vi "SBA-5_initialize.vi"(8 "error in (no error)":errorcluster, 9 "Valve control":bool=TRUE, 11 "VISA resource name":refnum<visa-resource-name>) -> (0 "error out":errorcluster, 3 "VISA resource name out":refnum<visa-resource-name>)   [LabVIEW 2016]
uses:
  <vilib>/Instr/_visa.llb/VISA Flush IO Buffer Mask.ctl
  <vilib>/Instr/_visa.llb/VISA Configure Serial Port (Instr).vi
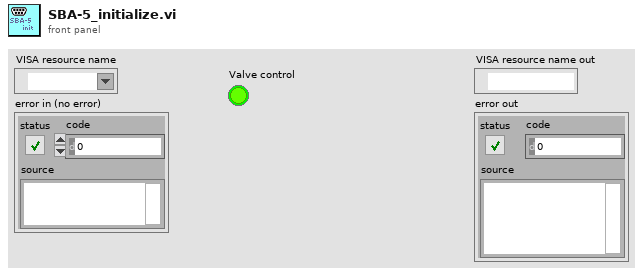
[diagram p1: front panel]
types:
  T1 = typedef "VISA Flush IO Buffer Mask.ctl" = u16
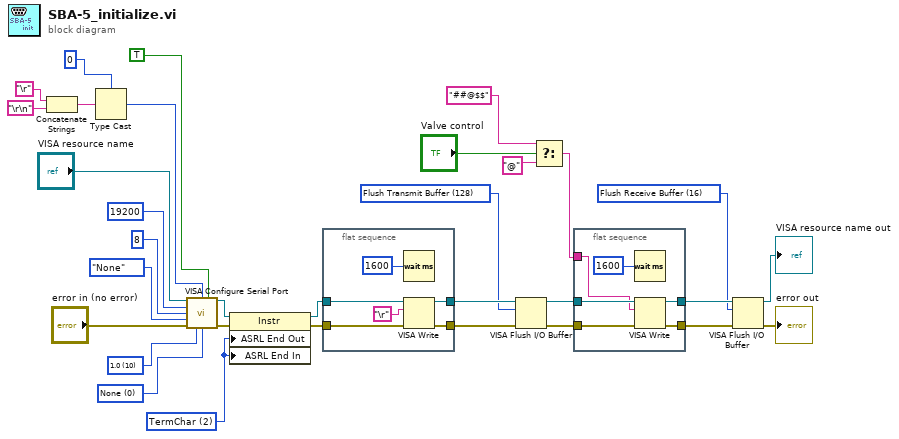
[diagram p0: block diagram]
diagram:
  w5 = T1 16 items=["Flush Receive Buffer"=16, "Write Transmit Buffer to Device"=32, "Flush Receive Buffer (No I/O)"=64, "Flush Transmit Buffer"=128] ("Mask")
  w11 = T1 128 items=["Flush Receive Buffer"=16, "Write Transmit Buffer to Device"=32, "Flush Receive Buffer (No I/O)"=64, "Flush Transmit Buffer"=128] ("Mask")
  w25 = u16 2 items=["None", "Last Bit", "TermChar", "Break"] ("Serial Settings:End Mode for Writes")
  w28 = u16 0 items=["None", "XON/XOFF", "RTS/CTS", "XON/XOFF & RTS/CTS", "DTR/DSR", "XON/XOFF & DTR/DSR"] ("flow control (0:none)")
  w29 = u16 10 items=["1.0"=10, "1.5"=15, "2.0"=20] ("stop bits (10: 1 bit)")
  n1 = Concatenate Strings("\r", "\r\n") -> (w10:string)
  n2 = Type Cast(type=u8 0, x=w10) -> (*(type *) &x=w7:u8)
  n3 = call-poly "VISA Configure Serial Port"("VISA resource name"="VISA resource name", "termination char\n(0xA = '\\n' = LF)"=w7, "Enable Termination\nChar (T)"=TRUE ("Enable Termination\nChar (T)"), "baud rate (9600)"=u32 19200 ("baud rate (19200)"), "data bits (8)"=u16 8, "parity (0:none)"=enum16{"None", "Odd", "Even", "Mark", "Space"}."None", "error in (no error)"="error in (no error)", "stop bits (10: 1 bit)"=w29, "flow control (0:none)"=w28) -> ("VISA resource name out"=w27:refnum<visa-resource-name>, "error out"=w26:errorcluster)  [unwired: 5 in]
  n4 = property class="Instr"(reference=w27, error in=w26, "ASRL End Out"=w25, "ASRL End In"=w25) -> (reference out=w24:refnum<visa-resource-name>, error out=w23:errorcluster)
  n5 = flat-sequence {
    tunnel: w24 -> [w38]
    tunnel: w23 -> [w37]
    tunnel: [w35] -> w19
    tunnel: [w34] -> w18
    frame #0 {
      n6 = Wait (ms)(milliseconds to wait=u32 1600) -> ()  [unwired: 1 out]
      n7 = VISA Write(VISA resource name=w38, write buffer="\r", error in (no error)=w37) -> (VISA resource name out=w35:refnum<visa-resource-name>, error out=w34:errorcluster)  [unwired: 1 out]
    }
  }
  n8 = VISA Flush I/O Buffer(VISA resource name=w19, mask (16)=w11, error in (no error)=w18) -> (VISA resource name out=w17:refnum<visa-resource-name>, error out=w16:errorcluster)
  n9 = Select(t="##@$$" ("write buffer"), s="Valve control", f="@") -> (s? t:f=w1:string)
  n10 = flat-sequence {
    tunnel: w17 -> [w44]
    tunnel: w16 -> [w43]
    tunnel: [w42] -> w13
    tunnel: [w41] -> w12
    tunnel: w1 -> [w39]
    frame #0 {
      n11 = Wait (ms)(milliseconds to wait=u32 1600) -> ()  [unwired: 1 out]
      n12 = VISA Write(VISA resource name=w44, write buffer=w39, error in (no error)=w43) -> (VISA resource name out=w41:refnum<visa-resource-name>, error out=w42:errorcluster)  [unwired: 1 out]
    }
  }
  n13 = VISA Flush I/O Buffer(VISA resource name=w12, mask (16)=w5, error in (no error)=w13) -> (VISA resource name out=→"VISA resource name out":refnum<visa-resource-name>, error out=→"error out":errorcluster)
